vi "#2 ON-OFF Led.vi"() -> ()   [LabVIEW 2013]
uses:
  <vilib>/LabVIEW Interface for Arduino/Type Defs/Pin Mode.ctl
  <vilib>/LabVIEW Interface for Arduino/LabVIEW Interface for Arduino.lvlib
panel:
  out "Boolean 2":bool
  in  "Boolean":bool
  in  "Digital I/O Pin (0)":u8
  in  "Pin Mode (Input)":T1
  in  "stop":bool
  in  "VISA resource":refnum<visa-resource-name>
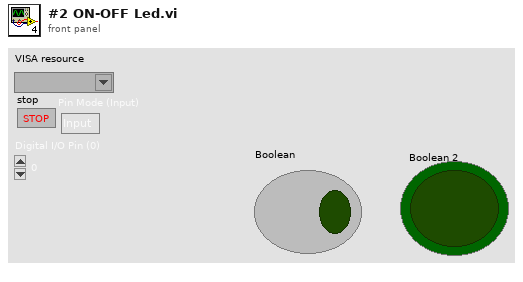
[diagram p1: front panel]
types:
  T1 = typedef "LabVIEW Interface for Arduino.lvlib/Pin Mode.ctl" = enum8{"Input", "Output"}
  T2 = typedef "LabVIEW Interface for Arduino.lvlib/Arduino Resource.ctl" = cluster{"VISA resource":refnum<visa-resource-name>, "Board Type":T3, "Connection Type":enum8{"USB / Serial"}, "Bytes Per Packet (15)":u8}
  T3 = typedef "LabVIEW Interface for Arduino.lvlib/Board Type.ctl" = enum16{"Uno", "Dimuelanove w/Atmega 328", "Mega 2560"}
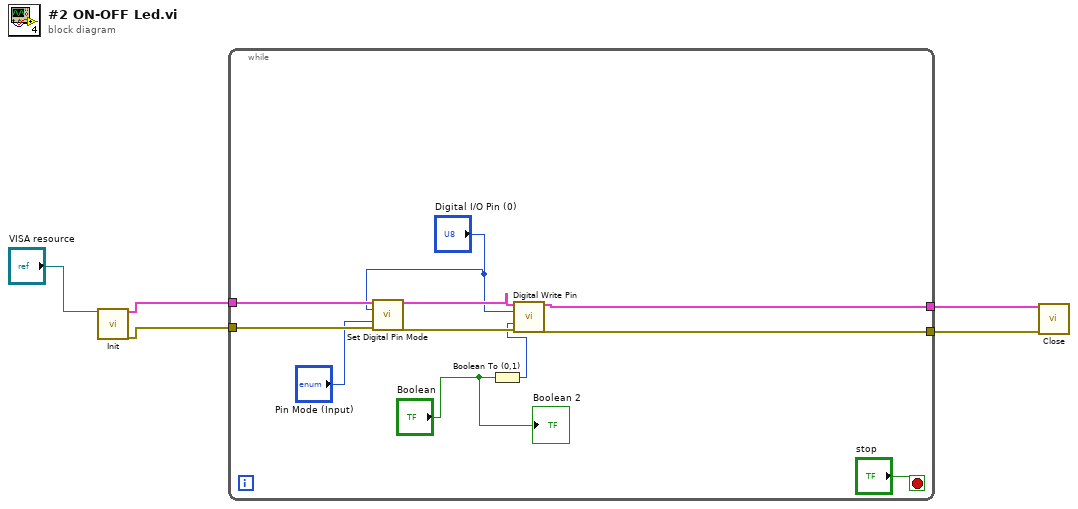
[diagram p0: block diagram]
diagram:
  n1 = call <vilib>:"Init.vi"("VISA resource"="VISA resource") -> ("Arduino Resource"=w5:T2, "error out"=w2:errorcluster)  [unwired: 17 in]
  n2 = while {
    tunnel: w5 -> [w16]
    tunnel: [w14] -> w4
    tunnel: [w13] -> w3
    tunnel: w2 -> [w11]
    stop <- "stop" stop-if-true
    n3 = call <vilib>:"Set Digital Pin Mode.vi"("Arduino Resource"=w16, "Digital I/O Pin"="Digital I/O Pin (0)", "Pin Mode (Input)"="Pin Mode (Input)", "error in"=w11) -> ("Arduino Resource"=w15:T2, "error out"=w12:errorcluster)  [unwired: 10 in]
    n4 = Boolean To (0,1)(Boolean="Boolean") -> (0, 1=w7:i16)
    n5 = call <vilib>:"Digital Write Pin.vi"("Arduino Resource"=w15, "Digital I/O Pin (0)"="Digital I/O Pin (0)", "Value (0)"=w7, "error in"=w12) -> ("Arduino Resource"=w14:T2, "error out"=w13:errorcluster)  [unwired: 10 in]
    "Boolean 2" <- "Boolean"
  }
  n6 = call <vilib>:"Close.vi"("Arduino Resource"=w4, "error in"=w3) -> ()  [unwired: 13 in, 1 out]
